vi "GetTrigger.vi"(7 "ModuleID":i32, 8 "error in (no error)":errorcluster, 11 "Infiniium in":refnum<class "Infiniium.lvclass">) -> (0 "error out":errorcluster, 3 "Infiniium out":refnum<class "Infiniium.lvclass">)   [LabVIEW 2014, in "ScopePlugins.lvlib" / "Infiniium.lvclass"]
uses:
  Infiniium.lvclass
  ScopePluginBaseClass/ScopePluginsBase.lvclass
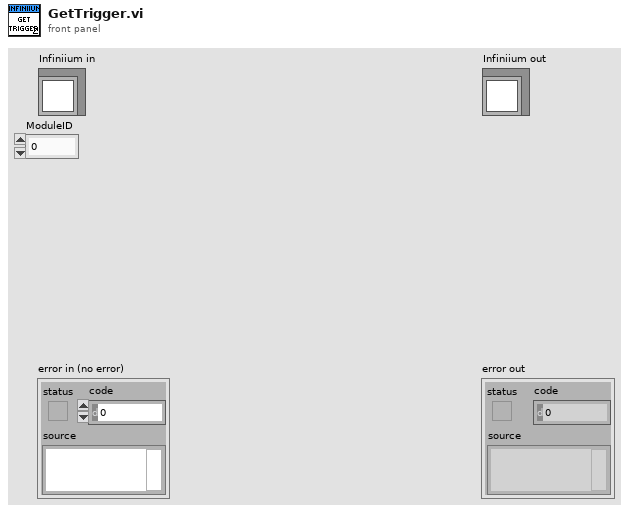
[diagram p1: front panel]
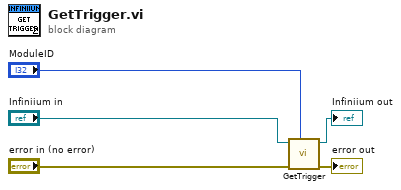
[diagram p0: block diagram]
diagram:
  n1 = call-parent "GetTrigger.vi"("ModuleID"="ModuleID", "error in (no error)"="error in (no error)", "ScopePluginsBase in"="Infiniium in") -> ("error out"=→"error out":errorcluster, "ScopePluginsBase out"=→"Infiniium out":refnum<class "Infiniium.lvclass">)  [unwired: 7 in]
